vi "Read Trigger Source.vi"(8 "error in (no error)":errorcluster, 11 "Camera in":refnum<class "Camera.lvclass">) -> (0 "error out":errorcluster, 2 "Trigger Source":string, 3 "Camera":refnum<class "Camera.lvclass">)   [LabVIEW 2020, in "Camera.lvclass"]
uses:
  Camera.lvclass
  Camera.lvclass/Camera.ctl
  bin/gindustrialcam_32-1.dll
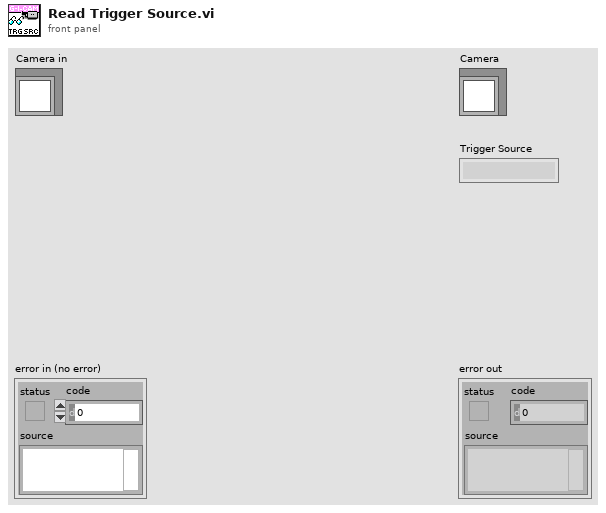
[diagram p1: front panel]
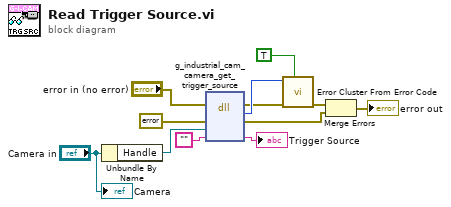
[diagram p0: block diagram]
diagram:
  n1 = Unbundle By Name("Camera in") -> ("Handle"=w7:refnum<data-value>)
  n2 = dll-call lib="C:/Workspace/SSDC/g-industrial-camera/LabVIEW/g_industrial_cam/bin/gindustrialcam_*-1.*" fn="g_industrial_cam_camera_get_trigger_source"(error in="error in (no error)", "err"=errorcluster {"status"=FALSE, "code"=0, "source"=""} ("error constant"), "edvr"=w7, "formats"="") -> (error out=w1:errorcluster, "Mg_Error"=w2:i32, "err"=w4:errorcluster, "formats"=→"Trigger Source":string)  [unwired: 3 in, 1 out]
  n3 = call <vilib>:"Error Cluster From Error Code.vi"("show call chain? (False)"=TRUE, "error in (no error)"=w1, "error code (0)"=w2) -> ("error out"=w3:errorcluster)  [unwired: 6 in]
  n4 = Merge Errors(w3, w4) -> (→"error out":errorcluster)
  "Camera" <- "Camera in"
